vi "EinlesenVonKalibrierung.vi"(8 "Error in":errorcluster, 10 "file path (use dialog)":path, 11 "EMTestCWS500N.lvclass":refnum<class "EMTestCWS500N.lvclass">) -> (0 "Error Out":errorcluster, 2 "String":string, 3 "EMTestCWS500N out":refnum<class "EMTestCWS500N.lvclass">)   [LabVIEW 2013, in "EMTestCWS500N.lvclass"]
uses:
  EMTestCWS500N.lvclass
  Main/controls/TestData.ctl
  Main/controls/TestStates.ctl
  lib/EMV-Test.lvlib
panel:
  out "Fortschritt":dbl(slide) scale=0.0..1.0
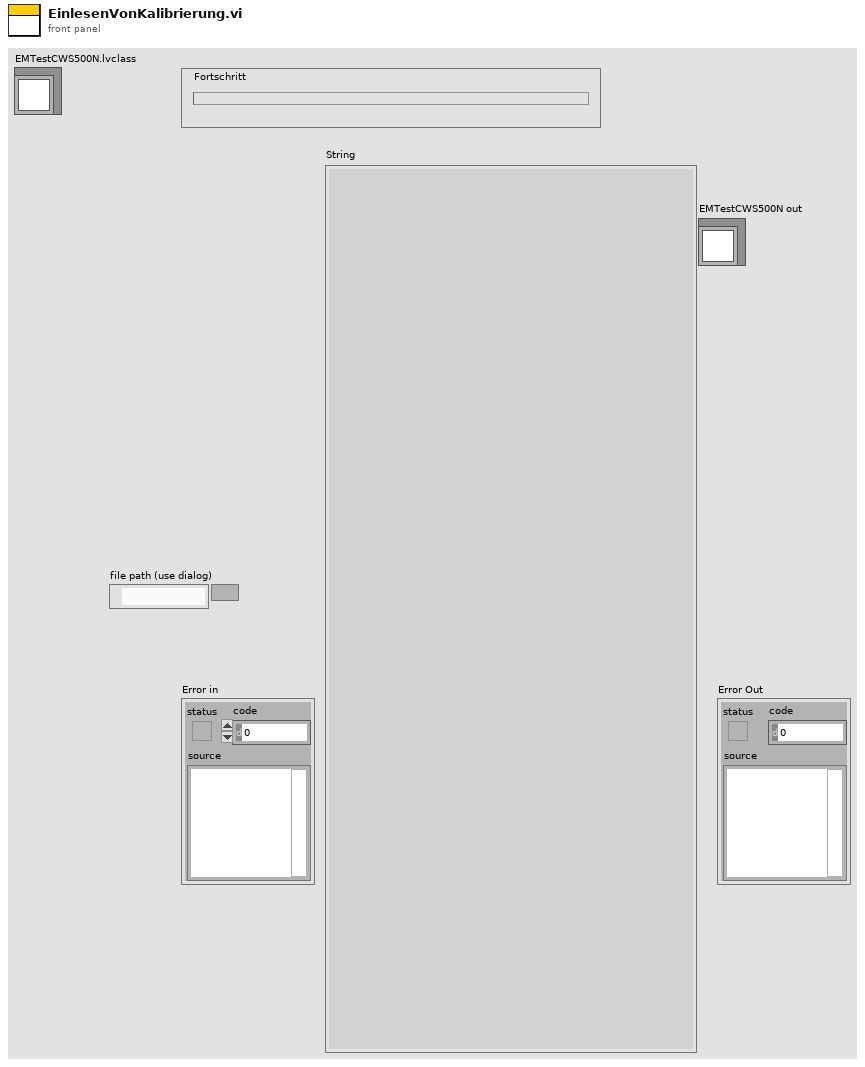
[diagram p1: front panel]
types:
  T1 = enum16{"open", "replace", "create", "open or create", "replace or create", "replace or create with confirmation"}
  T2 = typedef "EMV-Test.lvlib/TestData.ctl" = cluster{"commandlist":string, "line":i32, "last response":string, "timeout":i32, "wait":u32, "erfolgreich":bool, "next state":T3}
  T3 = typedef "EMV-Test.lvlib/TestStates.ctl" = enum16{"check for pressed Buttons", "pause", "vorgefertigter Test", "manueller Test", "respond to response", "error", "Start", "Initialise", "open connection", "evaluate line", "wait for Response", "wait", "catch error", "close Connection", "end", "empty buffer"}
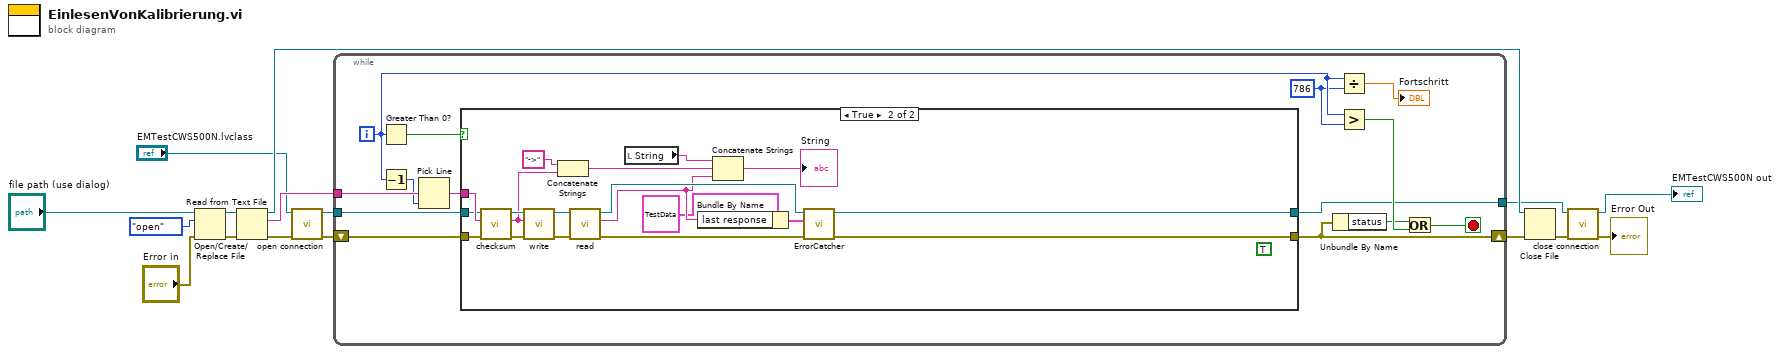
[diagram p0: block diagram]
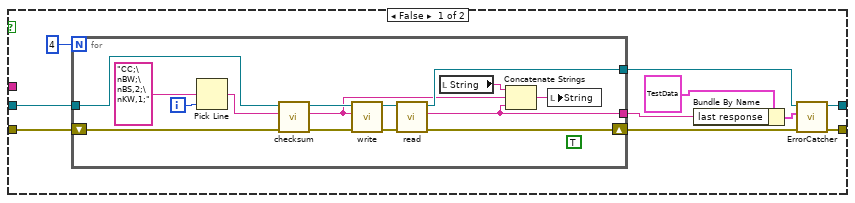
[diagram p2: hidden frame]
diagram:
  n1 = Open/Create/Replace File(file path (use dialog)="file path (use dialog)", error in="Error in", operation (0:open)=T1."open") -> (refnum out=w16:refnum<file>, error out=w15:errorcluster)  [unwired: 3 in, 1 out]
  n2 = Read from Text File(file (use dialog)=w16, error in=w15) -> (refnum out=w13:refnum<file>, text=w12:string, error out=w5:errorcluster)  [unwired: 2 in, 1 out]
  n3 = call-dynamic "open connection.vi"("error in (no error)"=w5, "EMTestCWS500N in"="EMTestCWS500N.lvclass") -> ("error out"=w3:errorcluster, "EMTestCWS500N out"=w4:refnum<class "EMTestCWS500N.lvclass">)  [unwired: 8 in]
  n4 = while {
    tunnel: w12 -> [w30]
    shift-right: [w21] -> w11
    shift-left: w3 -> [w22]
    tunnel: w4 -> [w27]
    tunnel: [w23] -> w6
    i -> [w18]
    stop <- w24 stop-if-true
    w17 = 786 ("y")
    n5 = Greater Than 0?(x=w18) -> (x > 0?=w29:bool)
    n6 = Decrement(x=w18) -> (x-1=w20:i32)
    n7 = Pick Line(multi-line string=w30, line index=w20) -> (output string=w28:string)  [unwired: 1 in]
    n8 = case shown="True" w29 {
      tunnel: w28 -> [_ w72]
      tunnel: w22 -> [w40 w71]
      tunnel: w27 -> [w38 w68]
      tunnel: [w35 w61] -> w23
      tunnel: [w36 w56] -> w21
      frame False {
        n9 = for {
          N: 4 -> [_]
          shift-right: [w43] -> w37
          shift-left: w40 -> [w47]
          tunnel: w38 -> [w46]
          tunnel: [w44] -> w34
          tunnel: [w42] -> w32
          i -> [w55]
          (unwired) TRUE ("checksum")
          n10 = Pick Line(multi-line string="CC;\nBW;\nBS,2;\nKW,1;", line index=w55) -> (output string=w45:string)  [unwired: 1 in]
          n11 = call-dynamic "checksum.vi"("error in (no error)"=w47, "input"=w45, "EMTestCWS500N in"=w46) -> ("error out"=w49:errorcluster, "output"=w41:string, "EMTestCWS500N out"=w48:refnum<class "EMTestCWS500N.lvclass">)  [unwired: 6 in]
          n12 = call-dynamic "write.vi"("error in (no error)"=w49, "String to send"=w41, "EMTestCWS500N in"=w48) -> ("error out"=w51:errorcluster, "EMTestCWS500N out"=w50:refnum<class "EMTestCWS500N.lvclass">)  [unwired: 7 in]
          n13 = call-dynamic "read.vi"("error in (no error)"=w51, "EMTestCWS500N in"=w50) -> ("error out"=w43:errorcluster, "Return String"=w42:string, "EMTestCWS500N out"=w44:refnum<class "EMTestCWS500N.lvclass">)  [unwired: 7 in]
          n14 = local read "String"() -> (w53:string)
          n15 = Concatenate Strings(w53, w41, w42) -> (w52:string)
          n16 = local write "String"(w52) -> ()
        }
        n17 = Bundle By Name(cluster=T2 {"commandlist"="", "line"=0, "last response"="", "timeout"=0, "wait"=0, "erfolgreich"=FALSE, "next state"=enum."check for pressed Buttons"}, "last response"=w32) -> (w31:T2)
        n18 = call-dynamic "ErrorCatcher.vi"("error in (no error)"=w37, 10:w31, "EMTestCWS500N in"=w34) -> ("error out"=w36:errorcluster, "EMTestCWS500N out"=w35:refnum<class "EMTestCWS500N.lvclass">)  [unwired: 7 in]
      }
      frame True {
        (unwired) TRUE ("checksum")
        n19 = call-dynamic "checksum.vi"("error in (no error)"=w71, "input"=w72, "EMTestCWS500N in"=w68) -> ("error out"=w70:errorcluster, "output"=w63:string, "EMTestCWS500N out"=w69:refnum<class "EMTestCWS500N.lvclass">)  [unwired: 6 in]
        n20 = call-dynamic "write.vi"("error in (no error)"=w70, "String to send"=w63, "EMTestCWS500N in"=w69) -> ("error out"=w66:errorcluster, "EMTestCWS500N out"=w67:refnum<class "EMTestCWS500N.lvclass">)  [unwired: 7 in]
        n21 = Concatenate Strings("->" ("string"), w63) -> (w64:string)
        n22 = call-dynamic "read.vi"("error in (no error)"=w66, "EMTestCWS500N in"=w67) -> ("error out"=w60:errorcluster, "Return String"=w59:string, "EMTestCWS500N out"=w62:refnum<class "EMTestCWS500N.lvclass">)  [unwired: 7 in]
        n23 = local read "String"() -> (w73:string)
        n24 = Bundle By Name(cluster=T2 {"commandlist"="", "line"=0, "last response"="", "timeout"=0, "wait"=0, "erfolgreich"=FALSE, "next state"=enum."check for pressed Buttons"} ("Cluster"), "last response"=w59) -> (w57:T2)
        n25 = Concatenate Strings(w73, w64, w59) -> (→"String":string)
        n26 = call-dynamic "ErrorCatcher.vi"("error in (no error)"=w60, 10:w57, "EMTestCWS500N in"=w62) -> ("error out"=w56:errorcluster, "EMTestCWS500N out"=w61:refnum<class "EMTestCWS500N.lvclass">)  [unwired: 7 in]
      }
    }
    n27 = Unbundle By Name(w21) -> ("status"=w25:bool)
    n28 = Divide(x=w18, y=w17) -> (x/y=→"Fortschritt":dbl)
    n29 = Greater?(x=w18, y=w17) -> (0:w26:bool)
    n30 = Or(x=w25, y=w26) -> (x .or. y?=w24:bool)
  }
  n31 = Close File(refnum=w13, error in=w11) -> (error out=w8:errorcluster)  [unwired: 1 out]
  n32 = call-dynamic "close connection.vi"("error in (no error)"=w8, "EMTestCWS500N in"=w6) -> ("error out"=→"Error Out":errorcluster, "EMTestCWS500N out"=→"EMTestCWS500N out":refnum<class "EMTestCWS500N.lvclass">)  [unwired: 8 in]
